vi "GetRobotCorners.vi"(1 "botAngle (rad)":dbl=-9.817477042468104, 2 "botY (m)":dbl, 3 "botX (m)":dbl=0.04428) -> (0 "Corner Points (m)":cluster{dbl, dbl}[](array[cluster])=[{-0.6075593373971605, -0.11424853706560435}, {0.42441410041794647, -0.5417059310174096}, {0.6961193373971605, 0.11424853706560427}, {-0.33585410041794644, 0.5417059310174097}])   [LabVIEW 2015, in "Navigation2017.lvlib" / "SubVIs - Navigation2017.lvlib"]
doc: "Outputs a list of x,y coordinates (in meters) for the 4 corners of the robot, transformed by a given x,y amount and angle."
uses:
  SubVIs - Navigation2017.lvlib
  Navigation2017.lvlib
  Util - Navigation2017.lvlib
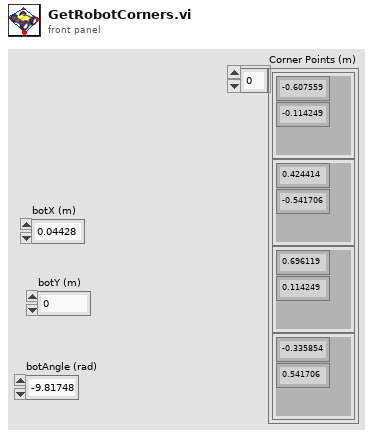
[diagram p1: front panel]
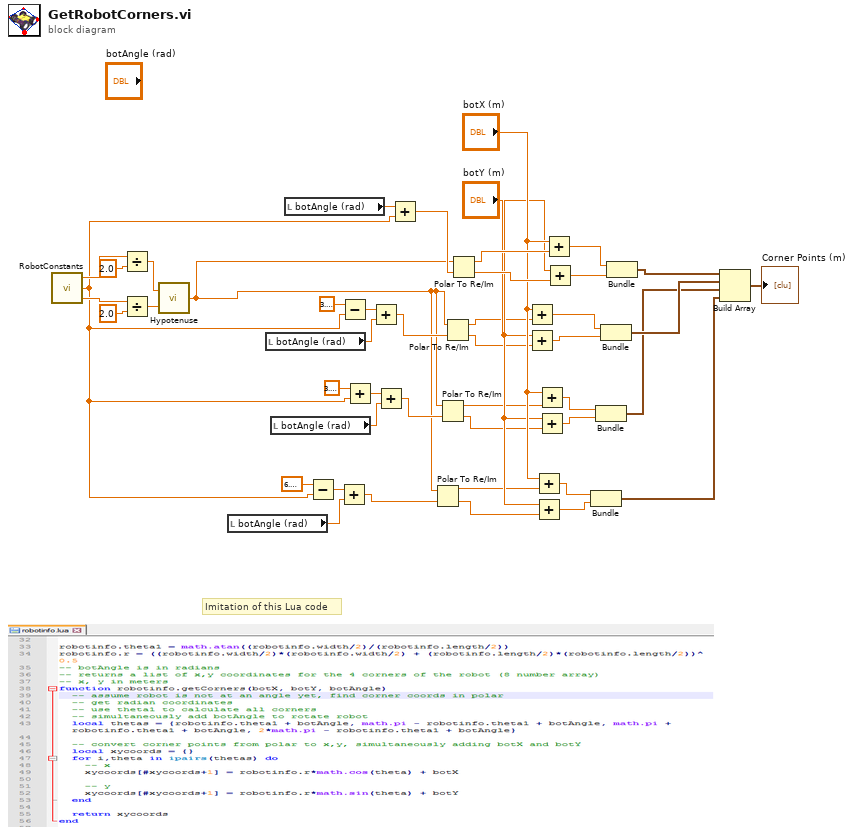
[diagram p0: block diagram]
diagram:
  # "Imitation of this Lua code"
  n1 = call "RobotConstants.vi"() -> ("Robot Width (m)"=w41:dbl, "atan((width/2) / (length/2))"=w24:dbl, "Robot Length (m)"=w40:dbl)  [unwired: 2 out]
  n2 = Divide(x=w41, y=2.0) -> (x/y=w44:dbl)
  n3 = Divide(x=w40, y=2.0) -> (x/y=w45:dbl)
  n4 = call "Hypotenuse.vi"("y"=w45, "x"=w44) -> ("r"=w20:dbl)
  n5 = local read "botAngle (rad)"() -> (w22:dbl)
  n6 = local read "botAngle (rad)"() -> (w33:dbl)
  n7 = local read "botAngle (rad)"() -> (w28:dbl)
  n8 = local read "botAngle (rad)"() -> (w38:dbl)
  n9 = Subtract(x=6.283185307179586, y=w24) -> (x-y=w23:dbl)
  n10 = Add(x=w23, y=w22) -> (x+y=w21:dbl)
  n11 = Subtract(x=3.141592653589793, y=w24) -> (x-y=w34:dbl)
  n12 = Add(x=3.141592653589793, y=w24) -> (x+y=w29:dbl)
  n13 = Add(x=w34, y=w33) -> (x+y=w32:dbl)
  n14 = Add(x=w29, y=w28) -> (x+y=w27:dbl)
  n15 = Add(x=w38, y=w24) -> (x+y=w36:dbl)
  n16 = Polar To Re/Im(2:w21, 3:w20) -> (0:w1:dbl, 1:w2:dbl)
  n17 = Polar To Re/Im(2:w27, 3:w20) -> (0:w3:dbl, 1:w4:dbl)
  n18 = Polar To Re/Im(2:w32, 3:w20) -> (0:w5:dbl, 1:w6:dbl)
  n19 = Polar To Re/Im(2:w36, 3:w20) -> (0:w15:dbl, 1:w17:dbl)
  n20 = Add(x="botX (m)", y=w6) -> (x+y=w14:dbl)
  n21 = Add(x="botY (m)", y=w5) -> (x+y=w13:dbl)
  n22 = Add(x="botX (m)", y=w2) -> (x+y=w10:dbl)
  n23 = Add(x="botY (m)", y=w1) -> (x+y=w9:dbl)
  n24 = Add(x="botX (m)", y=w4) -> (x+y=w12:dbl)
  n25 = Add(x="botY (m)", y=w3) -> (x+y=w11:dbl)
  n26 = Add(x="botX (m)", y=w17) -> (x+y=w18:dbl)
  n27 = Add(x="botY (m)", y=w15) -> (x+y=w16:dbl)
  n28 = Bundle(w10, w9) -> (w19:cluster{dbl, dbl})  [unwired: 1 in]
  n29 = Bundle(w12, w11) -> (w26:cluster{dbl, dbl})  [unwired: 1 in]
  n30 = Bundle(w14, w13) -> (w31:cluster{dbl, dbl})  [unwired: 1 in]
  n31 = Bundle(w18, w16) -> (w39:cluster{dbl, dbl})  [unwired: 1 in]
  n32 = Build Array(w39, w31, w26, w19) -> (→"Corner Points (m)":cluster{dbl, dbl}[])
